vi "数字量输出统计结果.vi"   [LabVIEW 2010]
uses:
  全局量/自动测试结果.vi
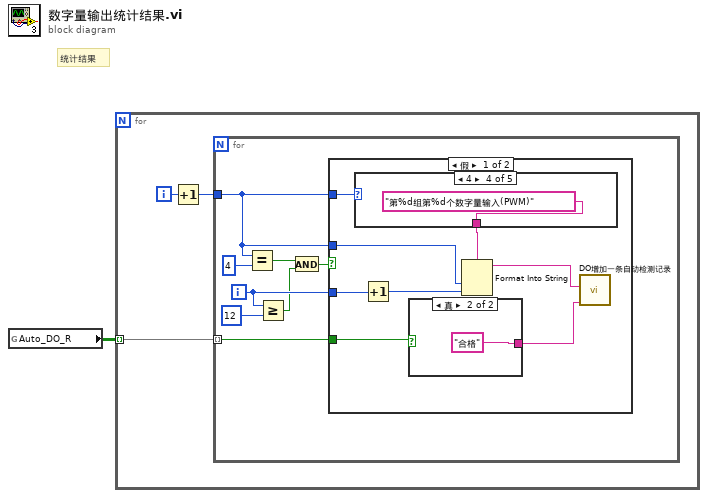
[diagram p0: block diagram]
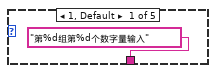
[diagram p2: hidden frame]
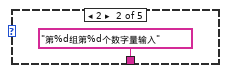
[diagram p3: hidden frame]
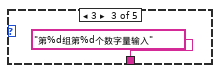
[diagram p4: hidden frame]
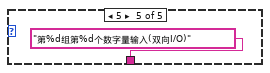
[diagram p5: hidden frame]
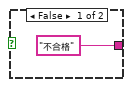
[diagram p6: hidden frame]
diagram:
  # "统计结果"
  n1 = global read "自动测试结果.vi" "Auto_DO_R"() -> (w1:bool[][])
  n2 = for {
    tunnel: w1 -> [w4] mode=indexing
    i -> [w3]
    n3 = Increment(x=w3) -> (x+1=w2:i32)
    n4 = for {
      tunnel: w4 -> [w12] mode=indexing
      tunnel: w2 -> [w5]
      i -> [w10]
      n5 = Equal?(x=w5, y=4) -> (x = y?=w8:bool)
      n6 = Greater Or Equal?(x=w10, y=12) -> (x >= y?=w7:bool)
      n7 = And(x=w8, y=w7) -> (x .and. y?=w6:bool)
      n8 = case shown="假" w6 {
        tunnel: w12 -> [w17 _]
        tunnel: w10 -> [w15 _]
        tunnel: w5 -> [w14 _]
        tunnel: w5 -> [w13 _]
        frame False {
          n9 = case shown="4" w13 {
            tunnel: ["第%d组第%d个数字量输入" "第%d组第%d个数字量输入" "第%d组第%d个数字量输入" "第%d组第%d个数字量输入(PWM)" "第%d组第%d个数字量输入(双向I/O)"] -> w20
            frame 1, Default {
            }
            frame 2 {
            }
            frame 3 {
            }
            frame 4 {
            }
            frame 5 {
            }
          }
          n10 = Increment(x=w15) -> (x+1=w19:i32)
          n11 = case shown="真" w17 {
            tunnel: ["不合格" "合格"] -> w16
            frame False {
            }
            frame True {
            }
          }
          n12 = Format Into String(format string=w20, w14, w19) -> (resulting string=w18:string)  [unwired: 2 in, 1 out]
          n13 = call "DO增加一条自动检测记录.vi"("测试结果"=w16, "测试内容"=w18) -> ()  [unwired: 10 in]
        }
        frame True {
        }
      }
    }
  }
